vi "PPR_TRAJECTORY_EXECUTE_ABS.vi"(8 "Init":bool, 10 "Max Wheel Speed M/S":dbl, 11 "End Pose ENG":T6={"TRANSLATION"={"X"=0.0, "Y"=0.0}, "ROTATION"={"VALUE"=0.0, "COS"=1.0, "SIN"=0.0}} {"ROTATION"."SIN" format="%13.4f"; "ROTATION"."COS" format="%13.4f"; "ROTATION"."VALUE" format="%13.4f"; "TRANSLATION"."Y" format="%14.3f"; "TRANSLATION"."X" format="%14.3f"}) -> (0 "AtReference":bool, 2 "Right Speed Dmd M/S":dbl, 3 "Left Speed Dmd M/S":dbl)   [LabVIEW 2019]
uses:
  <vilib>/Rock Robotics/WPI/ThirdParty/JAS_Junk/TrajLib/TypeDef/POSE2D.ctl
  <vilib>/Rock Robotics/WPI/ThirdParty/JAS_Junk/TrajLib/TypeDef/TRANSLATION2D.ctl
  <vilib>/Rock Robotics/WPI/ThirdParty/JAS_Junk/TrajLib/TypeDef/ROTATION2D.ctl
  <vilib>/Rock Robotics/WPI/ThirdParty/MJansen/PathPlanner/TypeDef/PathPlannerTrajectory.ctl
  <vilib>/Rock Robotics/WPI/ThirdParty/MJansen/PathPlanner/TypeDef/PathPlannerTrajectoryState.ctl
  <vilib>/Rock Robotics/WPI/ThirdParty/MJansen/PathPlanner/TypeDef/PathPlannerPathConstraints.ctl
  <vilib>/Rock Robotics/WPI/ThirdParty/JAS_Junk/TrajLib/VI/Util_GetTime_U32.vi
  <vilib>/Rock Robotics/WPI/ThirdParty/JAS_Junk/TrajLib/Rotation2d_GetRadians.vi
  <vilib>/Rock Robotics/WPI/ThirdParty/JAS_Junk/TrajLib/VI/Util_GetTime_U64.vi
  PPR_TRAJECTORY_GLOBALS.vi
  Diff_Drive_System/PPR_DRIVE_GLOBALS.vi
  <vilib>/Rock Robotics/WPI/ThirdParty/JAS_Junk/TrajLib/Trajectory_Library.lvlib
  <vilib>/Rock Robotics/WPI/ThirdParty/MJansen/PathPlanner/PathPlanner24.lvlib
panel:
  out "PathPlannerTrajectory":T1 {"States"."TargetHolonomicRotation"."SIN" format="%13.4f"; "States"."TargetHolonomicRotation"."COS" format="%13.4f"; "States"."TargetHolonomicRotation"."VALUE" format="%13.4f"; "States"."Heading"."SIN" format="%13.4f"; "States"."Heading"."COS" format="%13.4f"; "States"."Heading"."VALUE" format="%13.4f"; "States"."PositionMeters"."Y" format="%14.3f"; "States"."PositionMeters"."X" format="%14.3f"}
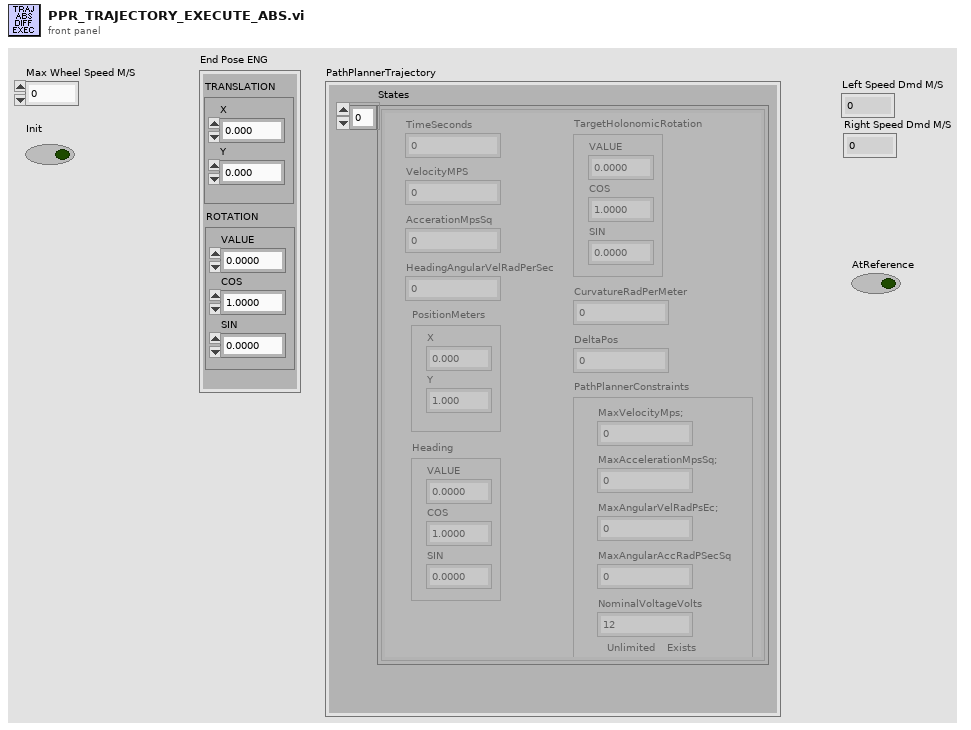
[diagram p1: front panel]
types:
  T1 = typedef "PathPlanner24.lvlib/PathPlannerTrajectory.ctl" = cluster{"States":T2[]}
  T2 = typedef "PathPlanner24.lvlib/PathPlannerTrajectoryState.ctl" = cluster{"TimeSeconds":dbl, "VelocityMPS":dbl, "AccerationMpsSq":dbl, "HeadingAngularVelRadPerSec":dbl, "PositionMeters":T3, "Heading":T4, "TargetHolonomicRotation":T4, "CurvatureRadPerMeter":dbl, "PathPlannerConstraints":T5, "DeltaPos":dbl}
  T3 = typedef "Trajectory_Library.lvlib/TRANSLATION2D.ctl" = cluster{"X":dbl, "Y":dbl}
  T4 = typedef "Trajectory_Library.lvlib/ROTATION2D.ctl" = cluster{"VALUE":dbl, "COS":dbl, "SIN":dbl}
  T5 = typedef "PathPlanner24.lvlib/PathPlannerPathConstraints.ctl" = cluster{"MaxVelocityMps;":dbl, "MaxAccelerationMpsSq;":dbl, "MaxAngularVelRadPsEc;":dbl, "MaxAngularAccRadPSecSq":dbl, "Exists":bool, "Unlimited":bool, "NominalVoltageVolts":dbl}
  T6 = typedef "Trajectory_Library.lvlib/POSE2D.ctl" = cluster{"TRANSLATION":T3, "ROTATION":T4}
  T7 = typedef "Trajectory_Library.lvlib/DIFF_DRIVE_KINEMATICS.ctl" = cluster{"TrackWidth_Meters":dbl}
  T8 = typedef "Trajectory_Library.lvlib/RAMSETE_EXE_TUNING.ctl" = cluster{"B":dbl, "Zeta":dbl, "X Tolerance M":dbl, "Y Tolerance M":dbl, "Heading Tolerance RAD":dbl, "Track Width M":dbl, "Max Speed M/S":dbl}
  T9 = typedef "Trajectory_Library.lvlib/RAMSETE.ctl" = cluster{"B":dbl, "Zeta":dbl, "poseTolerance":T6, "poseError":T6, "Enabled":bool}
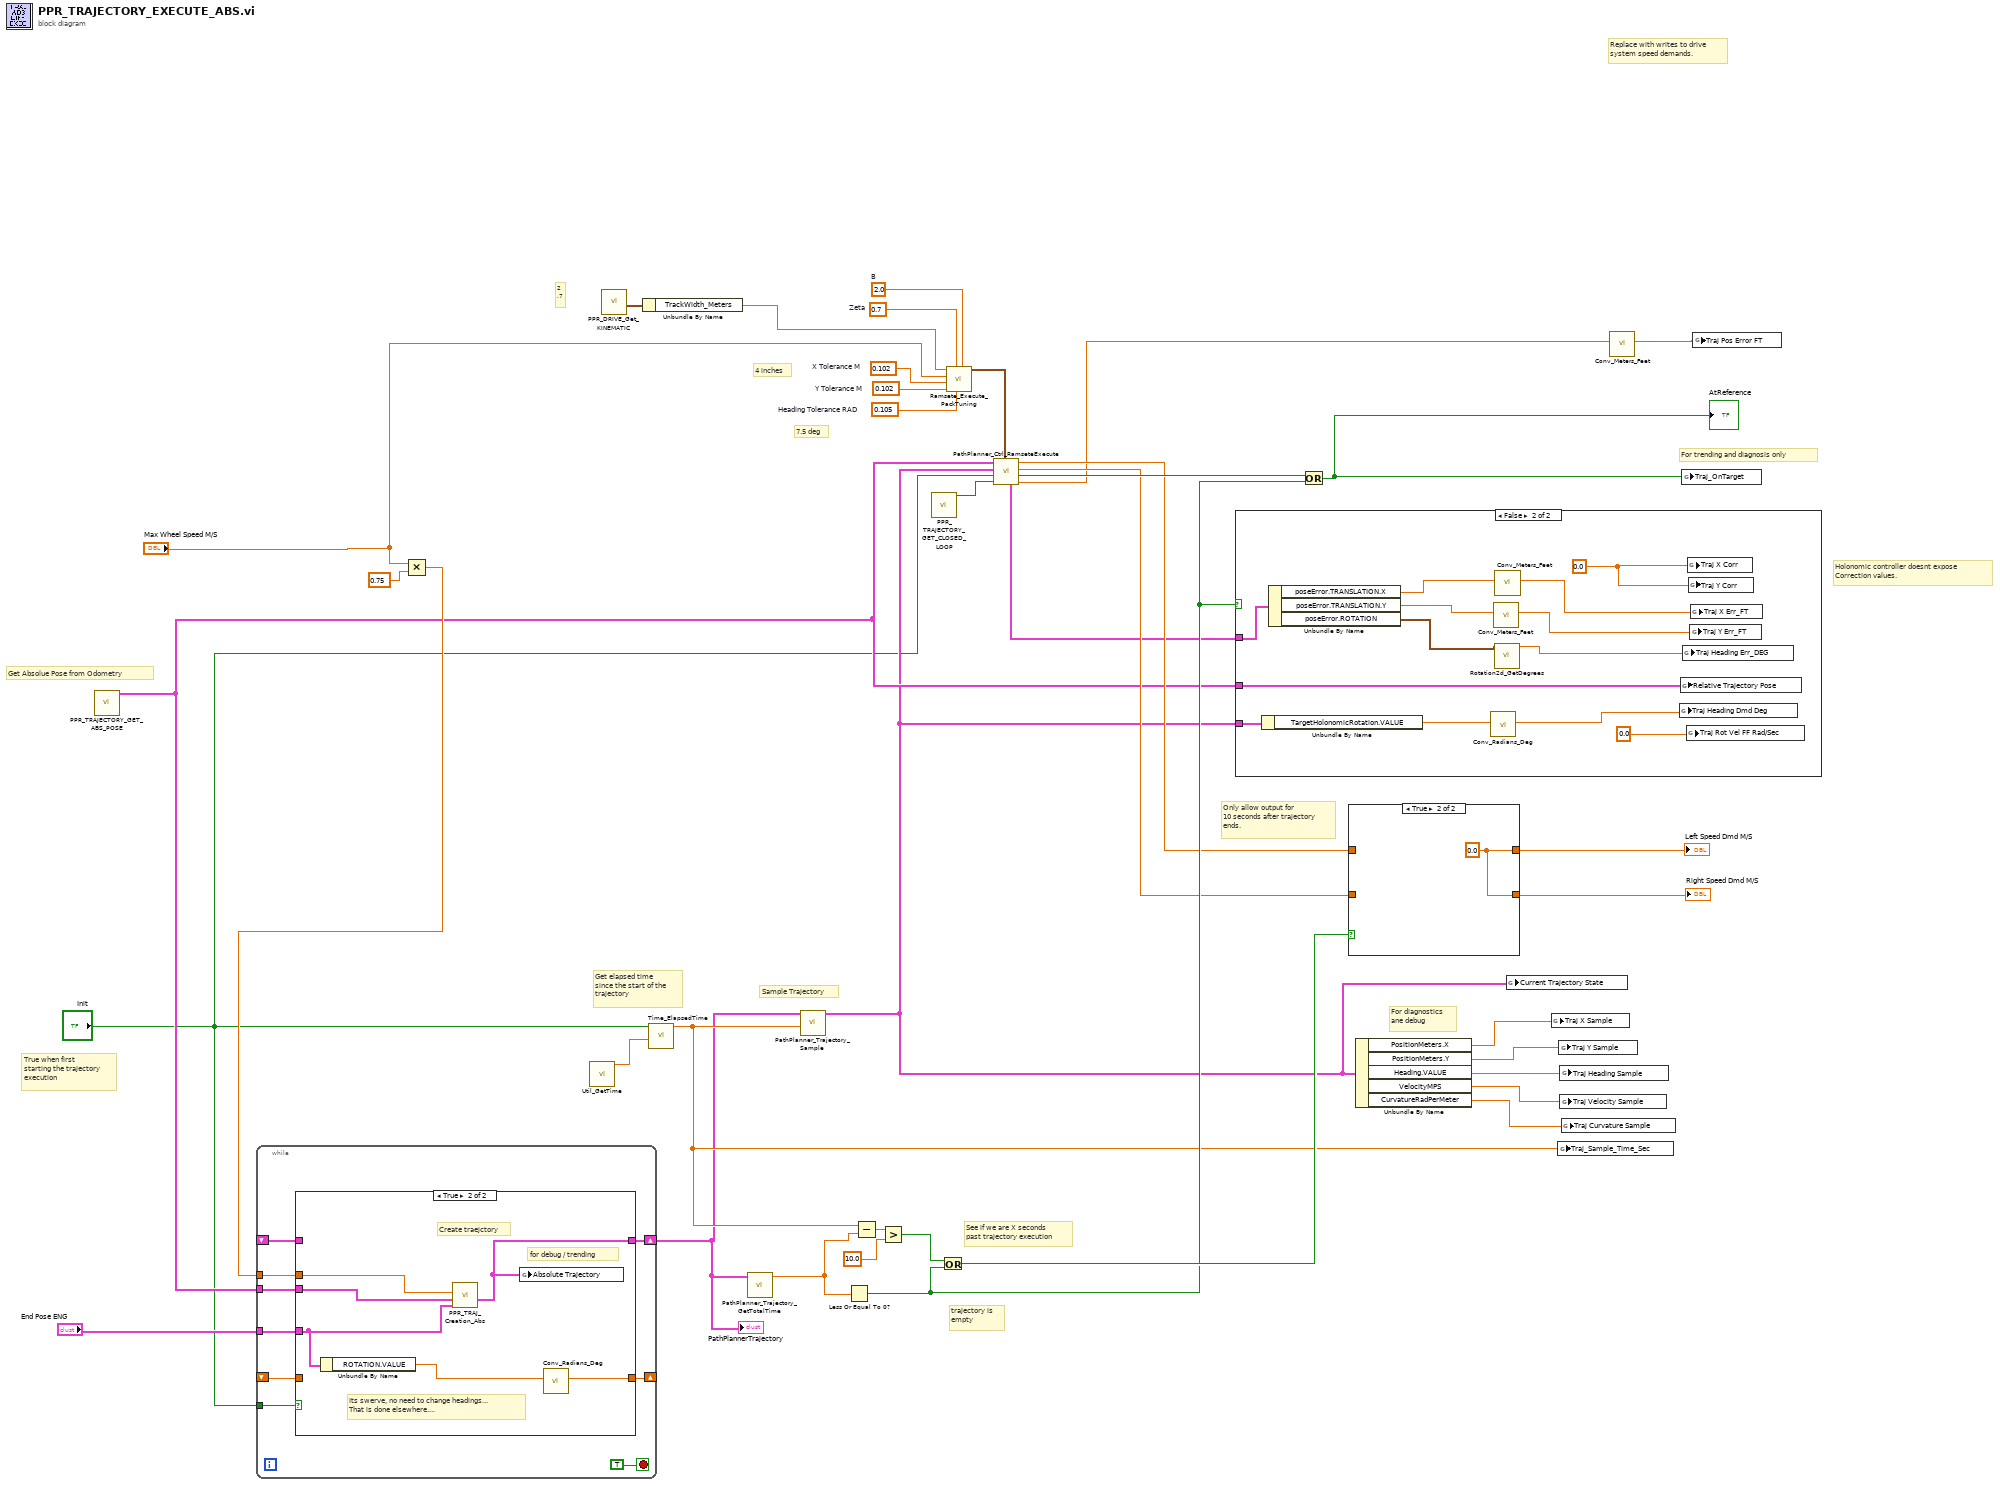
[diagram p0: block diagram]
diagram:
  w16 = 0.102  # X Tolerance M
  w17 = 0.102  # Y Tolerance M
  w18 = 0.7  # Zeta
  w19 = 0.105  # Heading Tolerance RAD
  w20 = 2.0  # B
  # "4 inches"
  # "7.5 deg"
  # "2\n.7"
  # "Replace with writes to drive\nsystem speed demands."
  # "trajectory is \nempty"
  # "True when first\nstarting the trajectory\nexecution"
  # "Get elapsed time\nsince the start of the\ntrajectory"
  # "Holonomic controller doesnt expose\nCorrection values."
  # "For trending and diagnosis only"
  # "For diagnostics\nane debug"
  # "Get Absolue Pose from Odometry"
  # "Sample Trajectory"
  # "See if we are X seconds \npast trajectory execution"
  # "Only allow output for\n10 seconds after trajectory\nends."
  n1 = call "PPR_TRAJECTORY_GET_ABS_POSE.vi"() -> ("Absolute Odometry Pose"=w5:T6)  [unwired: 11 in]
  n2 = Multiply(x="Max Wheel Speed M/S", y=0.75) -> (x*y=w23:dbl)
  n3 = while {
    tunnel: "Init" -> [w47]
    tunnel: w5 -> [w46]
    shift-right: [w45] -> w25
    shift-left: _ -> [w44]
    shift-right: [w43] -> _
    shift-left: _ -> [w42]
    tunnel: "End Pose ENG" -> [w41]
    tunnel: w23 -> [w40]
    stop <- TRUE stop-if-true
    n4 = case shown="True" w47 {
      tunnel: w46 -> [_ w52]
      tunnel: [w50 w53] -> w45
      tunnel: w44 -> [w50 _]
      tunnel: [w49 w55] -> w43
      tunnel: w42 -> [w49 _]
      tunnel: w41 -> [_ w56]
      tunnel: w40 -> [_ w51]
      frame False {
      }
      frame True {
        # "for debug / trending"
        # "Its swerve, no need to change headings...\nThat is done elsewhere...."
        # "Create traejctory"
        n5 = Unbundle By Name(w56) -> ("ROTATION.VALUE"=w54:dbl)
        n6 = call "PPR_TRAJ_Creation_Abs.vi"("End Pose  ENG"=w56, "Current Pose SI"=w52, "Max Velocity M/S"=w51) -> ("PathPlannerTrajectory"=w53:T1)  [unwired: 6 in, 2 out]
        n7 = global write "PPR_TRAJECTORY_GLOBALS.vi" "Absolute Trajectory"(w53) -> ()
        n8 = call <vilib>:"Conv_Radians_Deg.vi"("Radians"=w54) -> ("Degrees"=w55:dbl)  [unwired: 10 in]
      }
    }
  }
  "PathPlannerTrajectory" <- w25
  n9 = call <vilib>:"Util_GetTime.vi"() -> ("FPGA_Time_Seconds"=w37:dbl)  [unwired: 9 in, 2 out]
  n10 = call "PPR_DRIVE_Get_KINEMATIC.vi"() -> ("out DIFF_DRIVE_KINEMATICS"=w14:T7)  [unwired: 11 in]
  n11 = Unbundle By Name(w14) -> ("TrackWidth_Meters"=w13:dbl)
  n12 = call <vilib>:"Time_ElapsedTime.vi"("PassthroughTime_SEC"=w37, "Reset"="Init") -> ("Elapsed Time Sec"=w26:dbl)  [unwired: 9 in]
  n13 = call <vilib>:"PathPlanner_Trajectory_GetTotalTime.vi"("PathPlannerTrajectory"=w25) -> ("TotalTimeSeconds"=w24:dbl)  [unwired: 10 in]
  n14 = call <vilib>:"PathPlanner_Trajectory_Sample.vi"("Time"=w26, "PathPlannerTrajectory"=w25) -> ("PathPlannerState"=w4:T2)  [unwired: 9 in]
  n15 = Less Or Equal To 0?(x=w24) -> (x <= 0?=w27:bool)
  n16 = Subtract(x=w26, y=w24) -> (x-y=w39:dbl)
  n17 = Greater?(x=w39, y=10.0) -> (0:w30:bool)
  n18 = call "PPR_TRAJECTORY_GET_CLOSED_LOOP.vi"() -> ("AUTO_CLOSED_LOOP"=w2:bool)  [unwired: 11 in]
  n19 = Or(x=w30, y=w27) -> (x .or. y?=w29:bool)
  n20 = call <vilib>:"Ramsete_Execute_PackTuning.vi"("B"=w20, "Heading Tolerance RAD"=w19, "Zeta"=w18, "Y Tolerance M"=w17, "X Tolerance M"=w16, "Max Speed M/S"="Max Wheel Speed M/S", "Track Width M"=w13) -> ("RAMSETE_EXE_TUNING"=w21:T8)  [unwired: 4 in]
  n21 = call <vilib>:"PathPlanner_Ctrl_RamseteExecute.vi"("RAMSETE_EXE_TUNING SI"=w21, "Enabled"=w2, "Reset"="Init", "PathPlannerState"=w4, "Current Pose SI"=w5) -> ("Position Error M"=w6:dbl, "At Reference"=w15:bool, "Right Speed Dmd M/S"=w10:dbl, "Left Speed Dmd M/S"=w12:dbl, "outRAMSETE"=w1:T9)  [unwired: 2 in]
  n22 = case shown="False" w27 {
    tunnel: w5 -> [_ w59]
    tunnel: w1 -> [_ w65]
    tunnel: w4 -> [_ w62]
    frame True {
    }
    frame False {
      w69 = 0.0 ("Y Corr")
      n23 = Unbundle By Name(w62) -> ("TargetHolonomicRotation.VALUE"=w61:dbl)
      n24 = Unbundle By Name(w65) -> ("poseError.TRANSLATION.X"=w64:dbl, "poseError.TRANSLATION.Y"=w63:dbl, "poseError.ROTATION"=w57:T4)
      n25 = call <vilib>:"Conv_Radians_Deg.vi"("Radians"=w61) -> ("Degrees"=w60:dbl)  [unwired: 10 in]
      n26 = call <vilib>:"Conv_Meters_Feet.vi"("Meters"=w63) -> ("Feet"=w68:dbl)  [unwired: 10 in]
      n27 = call <vilib>:"Rotation2d_GetDegrees.vi"("in ROTATION"=w57) -> ("AngleDegrees"=w58:dbl)  [unwired: 10 in]
      n28 = call <vilib>:"Conv_Meters_Feet.vi"("Meters"=w64) -> ("Feet"=w67:dbl)  [unwired: 10 in]
      n29 = global write "PPR_TRAJECTORY_GLOBALS.vi" "Traj Heading Dmd Deg"(w60) -> ()
      n30 = global write "PPR_TRAJECTORY_GLOBALS.vi" "Relative Trajectory Pose"(w59) -> ()
      n31 = global write "PPR_TRAJECTORY_GLOBALS.vi" "Traj Heading Err_DEG"(w58) -> ()
      n32 = global write "PPR_TRAJECTORY_GLOBALS.vi" "Traj Rot Vel FF Rad/Sec"(0.0 ("Traj Heading Dmd Deg")) -> ()
      n33 = global write "PPR_TRAJECTORY_GLOBALS.vi" "Traj X Corr"(w69) -> ()
      n34 = global write "PPR_TRAJECTORY_GLOBALS.vi" "Traj Y Corr"(w69) -> ()
      n35 = global write "PPR_TRAJECTORY_GLOBALS.vi" "Traj Y Err_FT"(w68) -> ()
      n36 = global write "PPR_TRAJECTORY_GLOBALS.vi" "Traj X Err_FT"(w67) -> ()
    }
  }
  n37 = Or(x=w15, y=w27) -> (x .or. y?=w28:bool)
  "AtReference" <- w28
  n38 = case shown="True" w29 {
    tunnel: w12 -> [w71 _]
    tunnel: [w71 w72] -> w11
    tunnel: w10 -> [w70 _]
    tunnel: [w70 w72] -> w9
    frame False {
    }
    frame True {
      w72 = 0.0 ("vX")
    }
  }
  "Left Speed Dmd M/S" <- w11
  "Right Speed Dmd M/S" <- w9
  n39 = Unbundle By Name(w4) -> ("PositionMeters.X"=w36:dbl, "PositionMeters.Y"=w35:dbl, "Heading.VALUE"=w34:dbl, "VelocityMPS"=w33:dbl, "CurvatureRadPerMeter"=w32:dbl)
  n40 = global write "PPR_TRAJECTORY_GLOBALS.vi" "Current Trajectory State"(w4) -> ()
  n41 = global write "PPR_TRAJECTORY_GLOBALS.vi" "Traj X Sample"(w36) -> ()
  n42 = global write "PPR_TRAJECTORY_GLOBALS.vi" "Traj_Sample_Time_Sec"(w26) -> ()
  n43 = global write "PPR_TRAJECTORY_GLOBALS.vi" "Traj Y Sample"(w35) -> ()
  n44 = global write "PPR_TRAJECTORY_GLOBALS.vi" "Traj Heading Sample"(w34) -> ()
  n45 = global write "PPR_TRAJECTORY_GLOBALS.vi" "Traj Velocity Sample"(w33) -> ()
  n46 = global write "PPR_TRAJECTORY_GLOBALS.vi" "Traj Curvature Sample"(w32) -> ()
  n47 = call <vilib>:"Conv_Meters_Feet.vi"("Meters"=w6) -> ("Feet"=w7:dbl)  [unwired: 10 in]
  n48 = global write "PPR_TRAJECTORY_GLOBALS.vi" "Traj_OnTarget"(w28) -> ()
  n49 = global write "PPR_TRAJECTORY_GLOBALS.vi" "Traj Pos Error FT"(w7) -> ()
